vi "Ex1_Add_Exec.vi"() -> ()   [LabVIEW 2013]
panel:
  out "standard output":string
  in  "working directory":path=path ""
  in  "command line":string
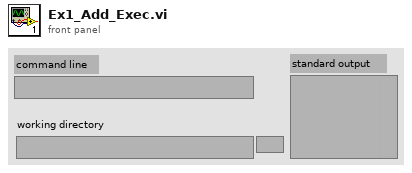
[diagram p1: front panel]
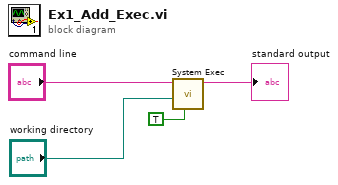
[diagram p0: block diagram]
diagram:
  n1 = call <vilib>:"System Exec.vi"("run minimized? (F)"=TRUE, "working directory"="working directory", "command line"="command line") -> ("standard output"=→"standard output":string)  [unwired: 5 in, 3 out]
